vi "Change Sonar I2C Address.vi"() -> ()   [LabVIEW 2011]
uses:
  <vilib>/LabVIEW Interface for Arduino/LabVIEW Interface for Arduino.lvlib
panel:
  in  "New Address":u8=165 format="%x"
  in  "Old Address":u8=112 format="%x"
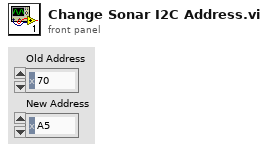
[diagram p1: front panel]
types:
  T1 = typedef "LabVIEW Interface for Arduino.lvlib/Arduino Resource.ctl" = cluster{"VISA resource":refnum<visa-resource-name>, "Board Type":T2, "Connection Type":enum8{"USB / Serial"}, "Bytes Per Packet (15)":u8}
  T2 = typedef "LabVIEW Interface for Arduino.lvlib/Board Type.ctl" = enum16{"Uno", "Dimuelanove w/Atmega 328", "Mega 2560"}
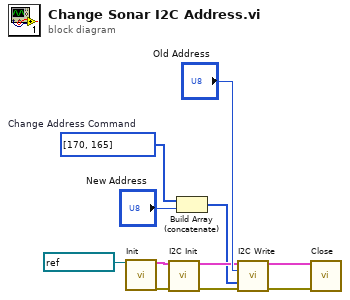
[diagram p0: block diagram]
diagram:
  w3 = u8[] [170, 165]  # Change Address Command
  n1 = call <vilib>:"Init.vi"("VISA resource"=refnum<visa-resource-name> "Arduino") -> ("Arduino Resource"=w11:T1, "error out"=w10:errorcluster)  [unwired: 17 in]
  n2 = call <vilib>:"I2C Init.vi"("Arduino Resource"=w11, "error in"=w10) -> ("Arduino Resource"=w5:T1, "error out"=w4:errorcluster)  [unwired: 12 in]
  n3 = Build Array (concatenate)(w3, "New Address") -> (w2:u8[])
  n4 = call <vilib>:"I2C Write.vi"("Arduino Resource"=w5, "Address (0)"="Old Address", "I2C Data Bytes"=w2, "error in"=w4) -> ("Arduino Resource"=w8:T1, "error out"=w7:errorcluster)  [unwired: 10 in]
  n5 = call <vilib>:"Close.vi"("Arduino Resource"=w8, "error in"=w7) -> ()  [unwired: 13 in, 1 out]
